vi "UpdateDialog.vi"(8 "error in (no error)":errorcluster, 10 "GameIn":refnum<class "Game.lvclass">, 11 "Highscore in":refnum<class "HighscoreDialog.lvclass">) -> (0 "error out":errorcluster, 2 "GameOut":refnum<class "Game.lvclass">, 3 "Highscore out":refnum<class "HighscoreDialog.lvclass">)   [LabVIEW 2019, in "RT_Game.lvlib" / "HighscoreDialog.lvclass"]
uses:
  HighscoreDialog/HighscoreDialog.lvclass
  C:/Users/FreshBob/Dropbox/VIs/myRIO_GameConsole/RT/RT_Game/GameObject/GameObject.lvclass
  Game/Game.lvclass
  GameObject/GameObject.lvclass/GameObject.ctl
  GameObject/Read IsActive.vi
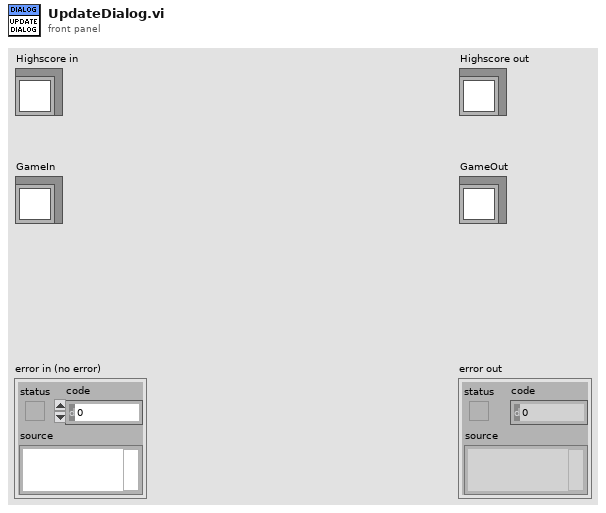
[diagram p1: front panel]
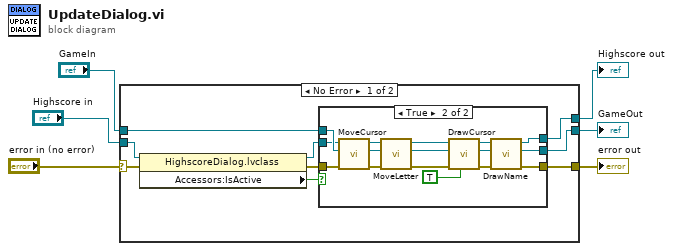
[diagram p0: block diagram]
diagram:
  n1 = case shown="No Error" "error in (no error)" {
    selector: "error in (no error)" -> [w15 w37]
    tunnel: [w12 w37] -> w5
    tunnel: [w13 w36] -> w3
    tunnel: "Highscore in" -> [w9 w36]
    tunnel: [w11 w35] -> w2
    tunnel: "GameIn" -> [w14 w35]
    frame No Error {
      n2 = property class="HighscoreDialog.lvclass"(reference=w9, error in=w15) -> (reference out=w8:refnum<class "HighscoreDialog.lvclass">, error out=w10:errorcluster, "Accessors:IsActive"=w7:bool)
      n3 = case shown="True" w7 {
        tunnel: w10 -> [w16 w34]
        tunnel: w14 -> [w17 w32]
        tunnel: w8 -> [w18 w31]
        tunnel: [w18 w22] -> w13
        tunnel: [w16 w20] -> w12
        tunnel: [w17 w19] -> w11
        frame False {
        }
        frame True {
          n4 = call "MoveCursor.vi"("error in (no error)"=w34, "GameIn"=w32, "Highscore in"=w31) -> ("error out"=w33:errorcluster, "Game out"=w28:refnum<class "Game.lvclass">, "Highscore out"=w29:refnum<class "HighscoreDialog.lvclass">)  [unwired: 6 in]
          n5 = call "MoveLetter.vi"("error in (no error)"=w33, "Game in"=w28, "Highscore in"=w29) -> ("error out"=w30:errorcluster, "Game out"=w25:refnum<class "Game.lvclass">, "Highscore out"=w26:refnum<class "HighscoreDialog.lvclass">)  [unwired: 6 in]
          n6 = call "DrawCursor.vi"("Visible?"=TRUE, "error in (no error)"=w30, "GameIn"=w25, "Highscore in"=w26) -> ("error out"=w27:errorcluster, "GameOut"=w21:refnum<class "Game.lvclass">, "Highscore out"=w23:refnum<class "HighscoreDialog.lvclass">)  [unwired: 5 in]
          n7 = call "DrawName.vi"("error in (no error)"=w27, "GameOut"=w21, "Highscore in"=w23) -> ("error out"=w20:errorcluster, "RT_Game.lvlib:Game.lvclass 2"=w19:refnum<class "Game.lvclass">, "Highscore out"=w22:refnum<class "HighscoreDialog.lvclass">)  [unwired: 6 in]
        }
      }
    }
    frame Error {
    }
  }
  "error out" <- w5
  "Highscore out" <- w3
  "GameOut" <- w2
